vi "Calculate Timeout in ms Based on Number of Bytes.vi"(11 "Number of Bytes":i32) -> (3 "Timeout (ms)":i32)   [LabVIEW 2013, in "TS.lvlib"]
uses:
  TS.lvlib
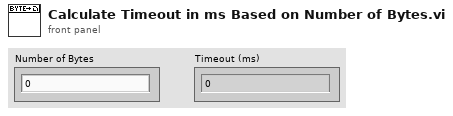
[diagram p1: front panel]
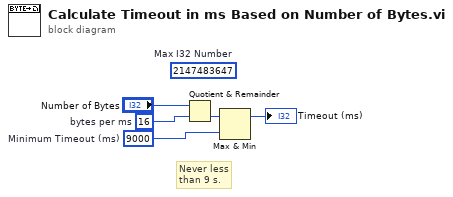
[diagram p0: block diagram]
diagram:
  (unwired) 2147483647  # Max I32 Number
  w2 = 16  # bytes per ms
  w5 = 9000  # Minimum Timeout (ms)
  # "Never less\nthan 9 s."
  n1 = Quotient & Remainder(x="Number of Bytes", y=w2) -> (floor(x/y)=w4:i32)  [unwired: 1 out]
  n2 = Max & Min(x=w4, y=w5) -> (max(x,y)=→"Timeout (ms)":i32)  [unwired: 1 out]
